vi "Reset Max-Min.vi"(8 "error in (no error)":errorcluster, 10 "Reset Max Min (True)":bool=TRUE, 11 "VISA resource name":refnum<visa-resource-name>) -> (0 "error out":errorcluster, 3 "VISA resource name out":refnum<visa-resource-name>)   [LabVIEW 2015, in "Lake Shore 372.lvlib"]
doc: "Resets Min/Max function for all channels."
uses:
  <instrlib>/Lake Shore 372/Lake Shore 372.lvlib
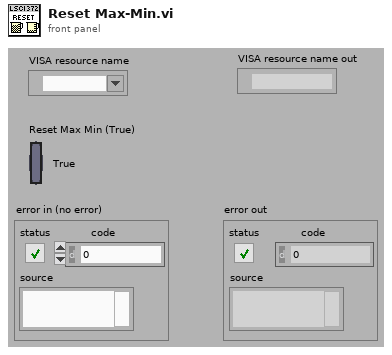
[diagram p1: front panel]
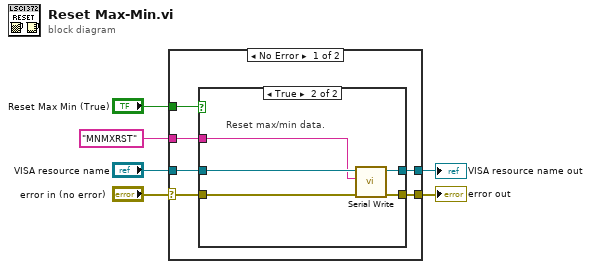
[diagram p0: block diagram]
diagram:
  n1 = case shown="No Error" "error in (no error)" {
    selector: "error in (no error)" -> [w7 w20]
    tunnel: "Reset Max Min (True)" -> [w12 _]
    tunnel: "VISA resource name" -> [w11 w21]
    tunnel: [w10 w21] -> w4
    tunnel: [w9 w20] -> w3
    tunnel: "MNMXRST" -> [w8 _]
    frame No Error {
      n2 = case shown="True" w12 {
        tunnel: w11 -> [w14 w19]
        tunnel: w7 -> [w13 w18]
        tunnel: [w14 w17] -> w10
        tunnel: [w13 w16] -> w9
        tunnel: w8 -> [_ w15]
        frame False {
          # "Do not reset max/min."
        }
        frame True {
          # "Reset max/min data."
          n3 = call <instrlib>:"Serial Write.vi"("error in (no error)"=w18, "Write Buffer (\"\")"=w15, "VISA resource name"=w19) -> ("error out"=w16:errorcluster, "VISA resource name out"=w17:refnum<visa-resource-name>)  [unwired: 6 in, 1 out]
        }
      }
    }
    frame Error {
    }
  }
  "VISA resource name out" <- w4
  "error out" <- w3
